vi "INI_Read LV INI Settings.vi"(8 "error in":errorcluster) -> (0 "error out":errorcluster, 3 "LabVIEW INI Settings":cluster{"Scripting":bool, "Private":bool})   [LabVIEW 2023]
doc: "Read LV ini file and determine is Scripting and Private settings are active."
uses:
  <resource>/dialog/lvconfig.llb/LV Config Read String.vi
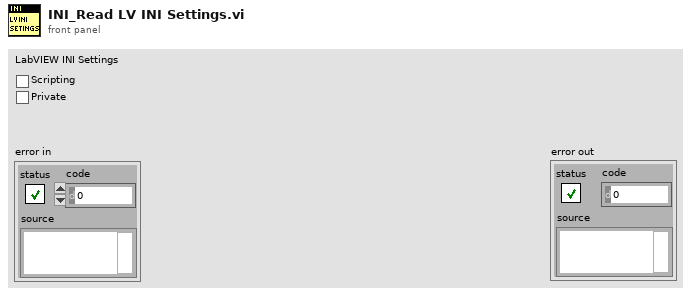
[diagram p1: front panel]
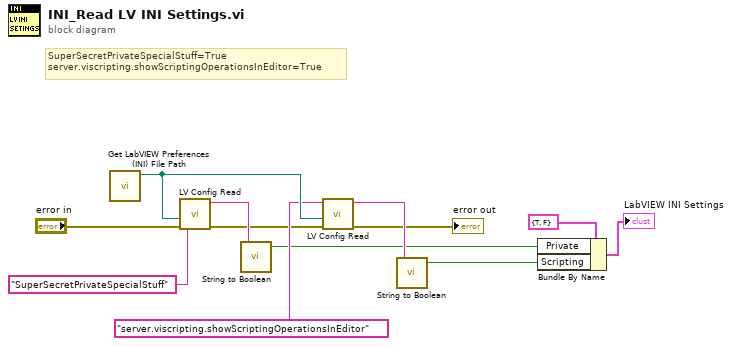
[diagram p0: block diagram]
diagram:
  # "SuperSecretPrivateSpecialStuff=True\nserver.viscripting.showScriptingOperationsInEditor=True"
  n1 = call <resource>:"Get LabVIEW Preferences (INI) File Path.vi"() -> ("LabVIEW Preferences (INI) File Path"=w10:path)  [unwired: 11 in]
  n2 = call-poly <resource>:"LV Config Read.vi"("error in"="error in", "config file path"=w10, "key"="SuperSecretPrivateSpecialStuff" ("regular expression")) -> ("error out"=w5:errorcluster, "value"=w7:string)  [unwired: 2 in, 1 out]
  n3 = call "String to Boolean.vi"("String"=w7) -> ("Boolean"=w1:bool)  [unwired: 4 in]
  n4 = call-poly <resource>:"LV Config Read.vi"("error in"=w5, "config file path"=w10, "key"="server.viscripting.showScriptingOperationsInEditor" ("regular expression")) -> ("error out"=→"error out":errorcluster, "value"=w6:string)  [unwired: 2 in, 1 out]
  n5 = call "String to Boolean.vi"("String"=w6) -> ("Boolean"=w2:bool)  [unwired: 4 in]
  n6 = Bundle By Name(cluster=cluster{"Scripting":bool, "Private":bool} {"Scripting"=TRUE, "Private"=FALSE} ("LabVIEW INI Settings"), "Private"=w1, "Scripting"=w2) -> (→"LabVIEW INI Settings":cluster{"Scripting":bool, "Private":bool})
